vi "Write-to-file-by-reference.vi"(8 "error in (no error)":errorcluster, 10 "Controls to save":refnum<vi>[](array[refnum]), 11 "SettingsFile in":refnum<class "SettingsFile.lvclass">) -> (0 "error out":errorcluster, 3 "SettingsFile out":refnum<class "SettingsFile.lvclass">)   [LabVIEW 2013, in "SettingsFile.lvlib" / "SettingsFile.lvclass"]
uses:
  SettingsFile.lvclass
  SettingsFile.lvclass/SettingsFile.ctl
  <vilib>/Utility/config.llb/Config Data RefNum.ctl
  Errors.ctl
  <vilib>/Utility/xml.llb/Write to XML File(string).vi
  <vilib>/Utility/config.llb/Write Key (String).vi
  <vilib>/Utility/config.llb/NI_LVConfig.lvlib
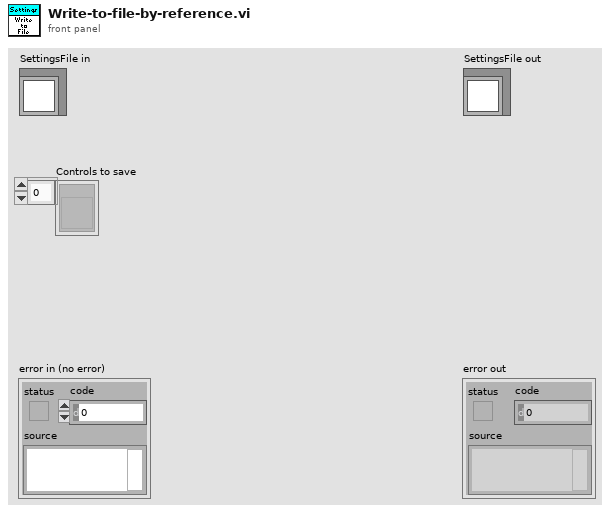
[diagram p1: front panel]
types:
  T1 = cluster{"Name":string, "Type":i16[], "Value":string}[]
  T2 = typedef "NI_LVConfig.lvlib/Config Data RefNum.ctl" = refnum<k1>
  T3 = typedef "SettingsFile.lvlib/SettingsFile.lvclass/Errors.ctl" = enum16{"Not implemented", "Command not recognized", "Invalid input", "No connection", "Timeout", "Invalid file type", "No file access"}
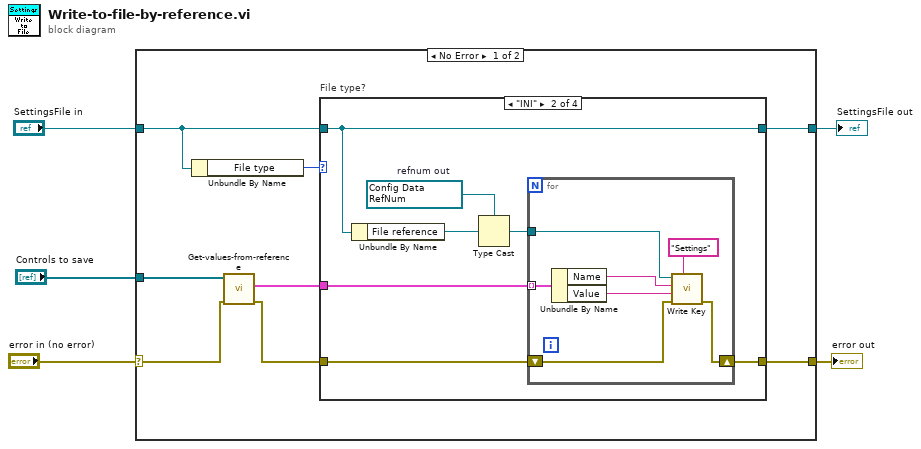
[diagram p0: block diagram]
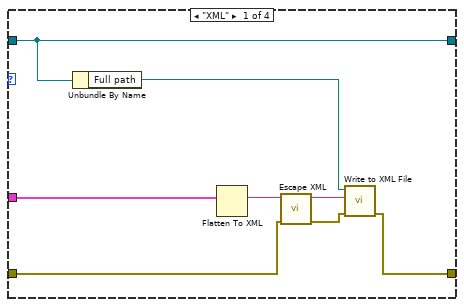
[diagram p2: hidden frame]
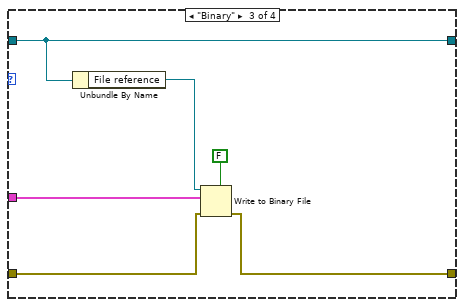
[diagram p3: hidden frame]
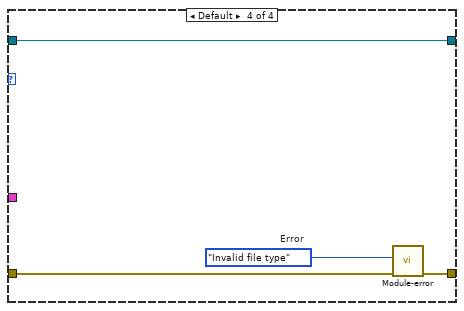
[diagram p4: hidden frame]
diagram:
  n1 = case shown="No Error" "error in (no error)" {
    selector: "error in (no error)" -> [w9 w47]
    tunnel: [w10 w47] -> w4
    tunnel: [w11 w46] -> w2
    tunnel: "SettingsFile in" -> [w12 w46]
    tunnel: "Controls to save" -> [w6 _]
    frame No Error {
      n2 = Unbundle By Name(w12) -> ("File type"=w13:enum16{"XML", "INI", "Binary"})
      n3 = call "Get-values-from-reference.vi"("error in (no error)"=w9, "Controls to save in"=w6) -> ("error out"=w8:errorcluster, "Values"=w7:T1)  [unwired: 7 in, 1 out]
      n4 = case "File type?" shown="\"INI\"" w13 {
        tunnel: w12 -> [w17 w28 w41 w45]
        tunnel: [w17 w28 w41 w45] -> w11
        tunnel: w8 -> [w16 w25 w38 w43]
        tunnel: [w15 w27 w37 w44] -> w10
        tunnel: w7 -> [w14 w26 w39 _]
        frame "XML" {
          n5 = Unbundle By Name(w17) -> ("Full path"=w18:path)
          n6 = Flatten To XML(anything=w14) -> (xml string=w20:string)
          n7 = call <vilib>:"Escape XML.vi"("error in (no error)"=w16, "XML String In"=w20) -> ("error out"=w19:errorcluster, "XML String Out"=w21:string)  [unwired: 8 in]
          n8 = call-poly <vilib>:"Write to XML File.vi"("error in (no error)"=w19, "XML Input"=w21, "XML File Path"=w18) -> ("error out"=w15:errorcluster)  [unwired: 6 in, 2 out]
        }
        frame "INI" {
          w24 = T2 refnum items=["config data"]  # refnum out
          n9 = Unbundle By Name(w28) -> ("File reference"=w23:refnum<file>)
          n10 = Type Cast(type=w24, x=w23) -> (*(type *) &x=w22:T2)
          n11 = for {
            tunnel: w26 -> [w34] mode=indexing
            shift-right: [w31] -> w27
            shift-left: w25 -> [w35]
            tunnel: w22 -> [w29]
            n12 = Unbundle By Name(w34) -> ("Name"=w33:string, "Value"=w32:string)
            n13 = call-poly <vilib>:"Write Key.vi"("section"="Settings", "error in (no error)"=w35, "value"=w32, "key"=w33, "refnum"=w29) -> ("error out"=w31:errorcluster)  [unwired: 4 in, 2 out]
          }
        }
        frame "Binary" {
          n14 = Unbundle By Name(w41) -> ("File reference"=w40:refnum<file>)
          n15 = Write to Binary File(file (use dialog)=w40, data=w39, error in=w38, 5:FALSE) -> (error out=w37:errorcluster)  [unwired: 2 in, 2 out]
        }
        frame Default {
          w42 = Errors."Invalid file type"  # Error
          n16 = call "Module-error.vi"("error in (no error)"=w43, "Error"=w42) -> ("error out"=w44:errorcluster)  [unwired: 9 in]
        }
      }
    }
    frame Error {
    }
  }
  "error out" <- w4
  "SettingsFile out" <- w2
